vi "Move_3Wheel.vi"(8 "error in (no error)":errorcluster, 10 "Cluster":cluster{"UDmm)":dbl, "Vcmd":dbl}, 11 "KNR in":T1) -> (0 "error out":errorcluster, 3 "KNR out":T1)   [LabVIEW 2013]
uses:
  <userlib>/KNR OS 3.0 LabVIEW Toolkit/Type Definition/KNR3 Reference.ctl
  <userlib>/_FPGA Interface Advanced Tools/FPGA Interface Base/FPGA Interface Base.lvclass
  <userlib>/KNR OS 3.0 LabVIEW Toolkit/Type Definition/Resource.ctl
  <vilib>/Platform/TimedLoop/XDataNode/timing_clust.ctl
  <vilib>/Platform/TimedLoop/XDataNode/nitl_modes.ctl
  <vilib>/Platform/TimedLoop/XDataNode/wakeup.ctl
  Global.vi
  <vilib>/platform/TimedLoop/XDataNode/XDataNode.xnode
  <vilib>/Platform/TimedLoop/XDataNode/XDNodeRunTimeDep.lvlib
panel:
  out "Position":i32
  out "PWM":dbl[](graph)
  out "appended array":dbl[](array[numeric])
  out "dirN":i32[](array[numeric])
  out "speed":dbl[](graph)
  out "position":dbl[](graph)
  out "L.U_b":dbl
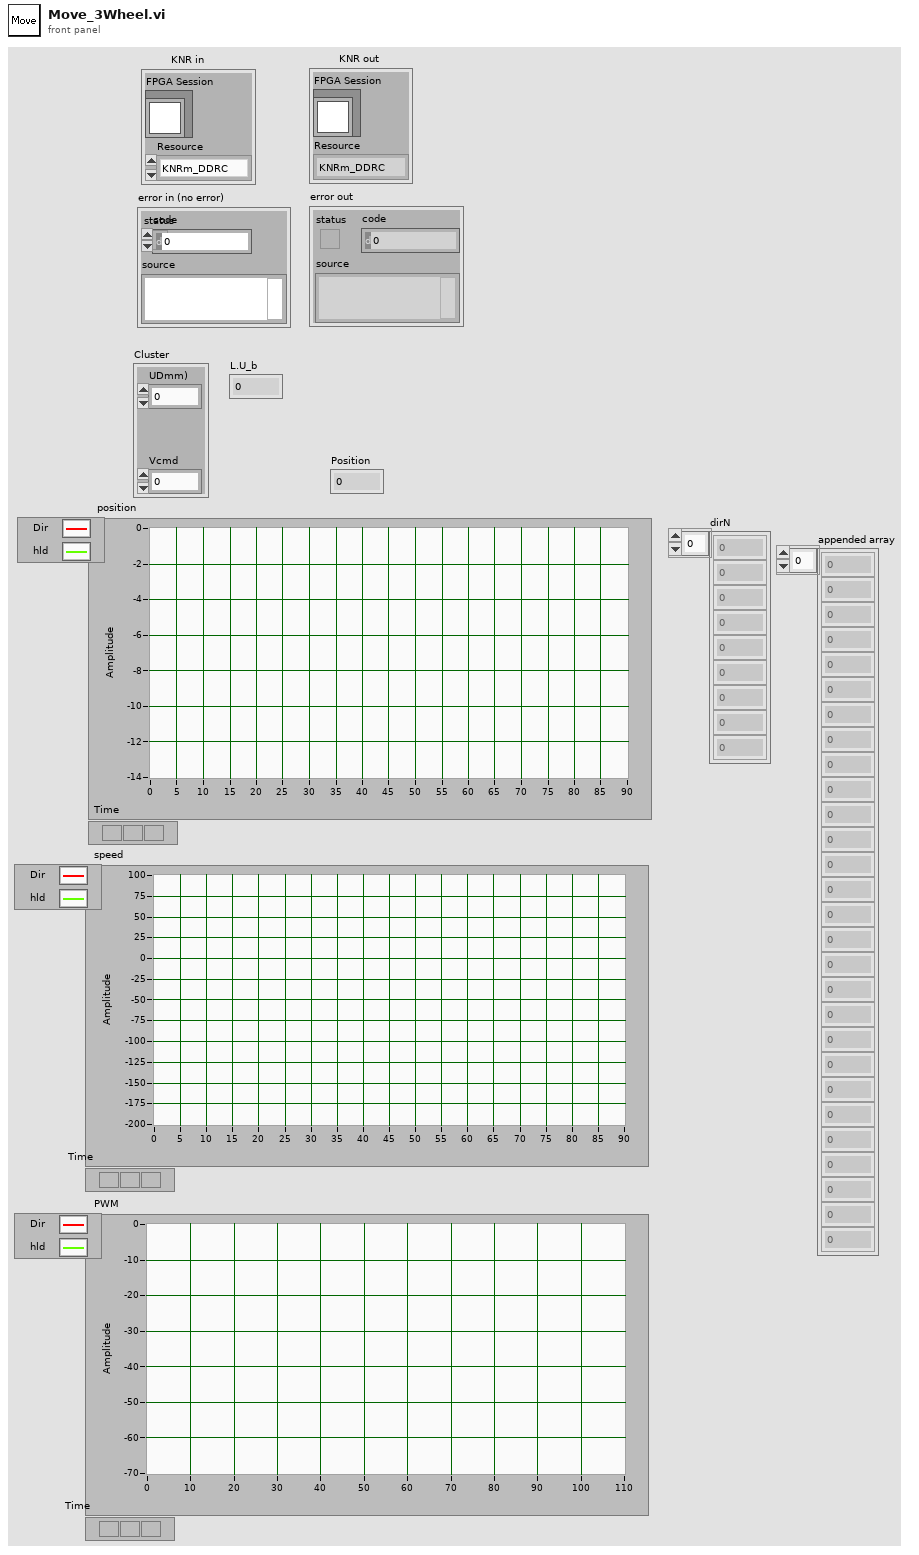
[diagram p1: front panel]
types:
  T1 = typedef "KNR3 Reference.ctl" = cluster{"FPGA Session":refnum<class "FPGA Interface Base.lvclass">, "Resource":T2}
  T2 = typedef "Resource.ctl" = enum16{"KNRm_DDRC", "KNRm_DDDD", "KNRm_DDDR", "KNRm_DDDC", "KNR"}
  T3 = cluster{"L":cluster{"enc":dbl, "enc_b":dbl, "Verr_b":dbl, "U_b":dbl}}
  T4 = typedef "DC Motor Port.ctl" = u16
  T5 = cluster{"MM2DEG":dbl, "PLS2DEG":dbl, "Ts":dbl, "Tcnt":i32, "fs":i32, "Vmax":dbl, "Jmax":dbl, "N_Delay":i32, "C_port":T4, "KNRPLS":dbl}
  T6 = cluster{"Ts":dbl, "deg":dbl, "V":dbl, "A":dbl, "J":dbl, "Lest":dbl, "dirN":i32[], "dirT":dbl[], "L":dbl[], "revgain":dbl}
  T7 = typedef "XDNodeRunTimeDep.lvlib/timing_clust.ctl" = cluster{"Expected End [f-1]":u64, "Actual End [f-1]":u64, "Finished Late? [f-1]":bool, "Expected End [i-1]":u64, "Actual End [i-1]":u64, "Finished Late? [i-1]":bool, "Expected Start [i]":u64, "Actual Start [i]":u64, "Expected Start [f]":u64, "Actual Start [f]":u64, "Source Name":string, "Structure Name":string, "Period":i64, "Deadline":i64, "Offset":i64, "Start":i64, "Priority":i32, "Timeout":i32, "Mode":T8, "Wakeup Reason":T9, "Error":errorcluster, "Source Type":string, "Secondary Source Type":string, "Global End Time":u64, "Global Start Time":u64, "Frame Duration":u64, "Iteration Duration":u64, "Assigned CPU":i32, "I/O Scan Engine Mode":u32}
  T8 = typedef "XDNodeRunTimeDep.lvlib/nitl_modes.ctl" = enum32{"No Change", "Process missed periods, maintain original phase", "Discard missed periods, maintain original phase", "Process missed periods, ignore original phase", "Discard missed periods, ignore original phase"}
  T9 = typedef "XDNodeRunTimeDep.lvlib/wakeup.ctl" = enum32{"Normal", "Aborted", "Asynchronous wakeup", "Timing source error", "Timed loop error", "Timeout"}
  T10 = cluster{"L":cluster{"Enc":dbl, "Enc_b":dbl, "Verr_b":dbl, "U_b":dbl}}
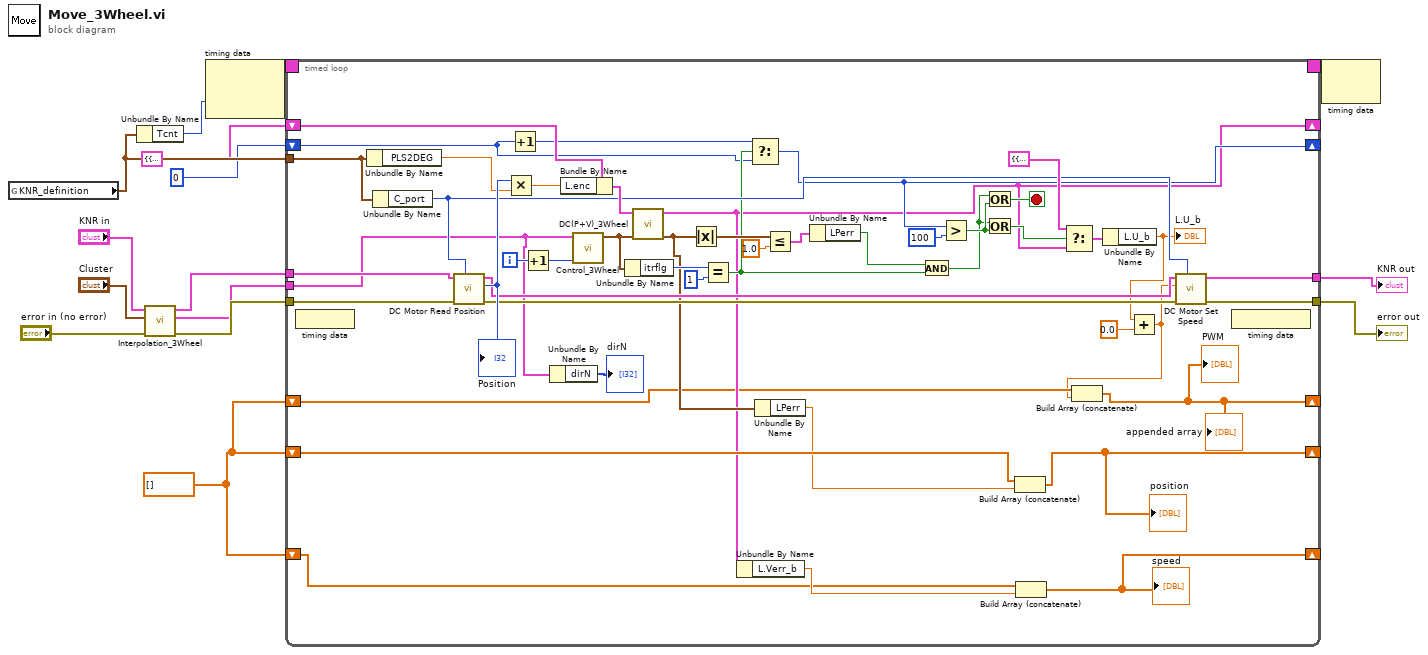
[diagram p0: block diagram]
diagram:
  w1 = dbl[] []
  n1 = global read "Global.vi" "KNR_definition"() -> (w7:T5)
  n2 = Unbundle By Name(w7) -> ("Tcnt"=w8:i32)
  n3 = call "Interpolation_3Wheel.vi"("error in (no error)"="error in (no error)", "Cluster"="Cluster", "KNR in"="KNR in") -> ("error out"=w10:errorcluster, "output cluster"=w9:T6, "KNR out"=w11:T1)  [unwired: 6 in]
  n4 = node-c288(w8) -> (w15:T7)  [unwired: 1 in]
  n5 = timed-loop {
    timing: w15 -> [_]
    timing-out: [_] -> w14
    tunnel: w11 -> [w63]
    tunnel: w10 -> [w62]
    tunnel: [w47] -> w4
    tunnel: [w46] -> w5
    tunnel: w9 -> [w21]
    tunnel: w7 -> [w43]
    shift-right: [w19] -> _
    shift-left: T3 {"L"={"enc"=0.0, "enc_b"=0.0, "Verr_b"=0.0, "U_b"=0.0}} ("control") -> [w57]
    shift-right: [w35] -> _
    shift-left: 0 -> [w38]
    shift-right: [w28] -> _
    shift-left: w1 -> [w29]
    shift-right: [w24] -> _
    shift-left: w1 -> [w25]
    shift-right: [w17] -> _
    shift-left: w1 -> [w18]
    i -> [w58]
    stop <- w40 stop-if-true
    n6 = node-c288() -> ()  [unwired: 1 in]
    n7 = Unbundle By Name(w43) -> ("PLS2DEG"=w48:dbl)
    n8 = Unbundle By Name(w43) -> ("C_port"=w42:T4)
    n9 = call <userlib>:"DC Motor Read Position.vi"("Port (DS1)"=w42, "error in (no error)"=w62, "KNR in"=w63) -> ("error out"=w44:errorcluster, "Position"=w61:i32, "KNR out"=w45:T1)  [unwired: 6 in]
    "Position" <- w61
    n10 = Multiply(x=w61, y=w48) -> (x*y=w49:dbl)
    n11 = Increment(x=w38) -> (x+1=w37:i32)
    n12 = Increment(x=w58) -> (x+1=w31:i32)
    n13 = Unbundle By Name(w21) -> ("dirN"=→"dirN":i32[])
    n14 = Bundle By Name(cluster=w57, "L.enc"=w49) -> (w56:T3)
    n15 = call "Control_3Wheel.vi"("cnt"=w31, "input"=w21) -> ("CMD"=w51:cluster{"Tcmd":dbl, "Ocmd":dbl, "itrflg":i32})  [unwired: 8 in]
    n16 = Unbundle By Name(w51) -> ("itrflg"=w53:i32)
    n17 = call "DC(P+V)_3Wheel.vi"("CMD"=w51, "control"=w56) -> ("output cluster 2"=w30:cluster{"LPerr":dbl}, "output cluster"=w19:T10)  [unwired: 8 in]
    n18 = Absolute Value(x=w30) -> (abs(x)=w55:cluster{"LPerr":dbl})
    n19 = Equal?(x=w53, y=1) -> (x = y?=w41:bool)
    n20 = Unbundle By Name(w19) -> ("L.Verr_b"=w26:dbl)
    n21 = Select(t=w37, s=w41, f=w38) -> (s? t:f=w35:i32)
    n22 = Unbundle By Name(w30) -> ("LPerr"=w27:dbl)
    n23 = Less Or Equal?(x=w55, y=1.0) -> (x <= y?=w54:cluster{"LPerr":bool})
    n24 = Unbundle By Name(w54) -> ("LPerr"=w32:bool)
    n25 = And(x=w32, y=w41) -> (x .and. y?=w33:bool)
    n26 = Greater?(x=w35, y=100) -> (0:w34:bool)
    n27 = Or(x=w33, y=w34) -> (x .or. y?=w40:bool)
    n28 = Or(x=w33, y=w34) -> (x .or. y?=w39:bool)
    n29 = Build Array (concatenate)(w29, w27) -> (w28:dbl[])
    "position" <- w28
    n30 = Build Array (concatenate)(w25, w26) -> (w24:dbl[])
    "speed" <- w24
    n31 = Select(t=T3 {"L"={"enc"=0.0, "enc_b"=0.0, "Verr_b"=0.0, "U_b"=0.0}} ("control"), s=w39, f=w19) -> (s? t:f=w52:T10)
    n32 = Unbundle By Name(w52) -> ("L.U_b"=w23:dbl)
    "L.U_b" <- w23
    n33 = Add(x=w23, y=0.0) -> (x+y=w16:dbl)
    n34 = Build Array (concatenate)(w18, w16) -> (w17:dbl[])
    "appended array" <- w17
    "PWM" <- w17
    n35 = call <userlib>:"DC Motor Set Speed.vi"("Port (DS1)"=w42, "error in (no error)"=w44, "Speed (+-100%)"=w16, "KNR in"=w45) -> ("error out"=w46:errorcluster, "KNR out"=w47:T1)  [unwired: 6 in]
    n36 = node-c288() -> ()  [unwired: 1 out]
  }
  "error out" <- w5
  "KNR out" <- w4
  n37 = node-c288(w14) -> ()  [unwired: 1 out]
